vi "Create Events.vi"(0 "Display State In":T2={"Nspeakers"=13, "actions"=[], "Wspeaker"=13, "hover"={"type"=enum."None", "index"=0}, "locked"=FALSE, "states"=[], "sel speak"=13, "selected"=refnum, "Events"={"Selection change"=refnum}}, 9 "Container State":T6, 11 "error in (no error)":errorcluster) -> (4 "Display State Out":T2={"Nspeakers"=13, "actions"=[], "Wspeaker"=13, "hover"={"type"=enum."None", "index"=0}, "locked"=FALSE, "states"=[], "sel speak"=13, "selected"=refnum, "Events"={"Selection change"=refnum}}, 8 "Events":T1, 15 "error out":errorcluster)   [LabVIEW 2015, in "SAC Config.xctl"]
uses:
  SAC Config.xctl
  <vilib>/_xctls/Container State.ctl
  State.vi
  Hover Data.ctl
  Hover Item.ctl
  Speaker State.ctl
  Events.ctl
  Selection changed.ctl
  <vilib>/_xctls/XControlSupport.lvlib
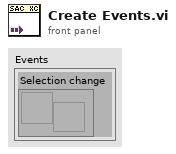
[diagram p1: front panel]
types:
  T1 = typedef "SAC Config.xctl/Events.ctl" = cluster{"Selection change":refnum<user-event>}
  T2 = typedef "SAC Config.xctl/State.vi" = cluster{"Nspeakers":i32, "actions":string[], "Wspeaker":i32, "hover":T3, "locked":bool, "states":T5[], "sel speak":i32, "selected":refnum<vi>, "Events":T1}
  T3 = typedef "SAC Config.xctl/Hover Data.ctl" = cluster{"type":T4, "index":i32}
  T4 = typedef "SAC Config.xctl/Hover Item.ctl" = enum16{"None", "Speaker"}
  T5 = typedef "SAC Config.xctl/Speaker State.ctl" = cluster{"cal":bool, "selected":bool}
  T6 = typedef "XControlSupport.lvlib/Container State.ctl" = cluster{"Indicator?":bool, "Run Mode?":bool, " Refnum":refnum<vi>}
  T7 = typedef "SAC Config.xctl/Selection changed.ctl" = cluster{"Value":i32[]}
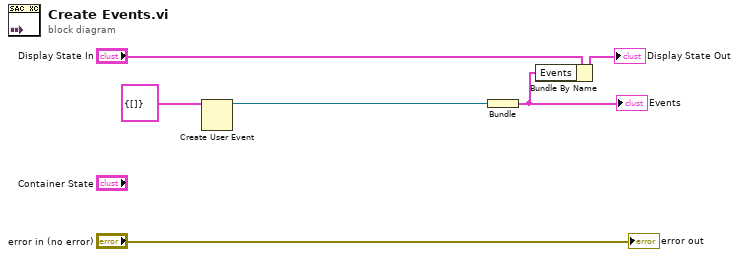
[diagram p0: block diagram]
diagram:
  n1 = Create User Event(user event datatype=T7 {"Value"=[]} ("Event Data")) -> (user event=w2:refnum<user-event>)  [unwired: 1 in, 1 out]
  n2 = Bundle("Event Data"=w2) -> (w1:cluster{"Event Data":refnum<user-event>})  [unwired: 1 in]
  "Events" <- w1
  n3 = Bundle By Name(cluster="Display State In", "Events"=w1) -> (→"Display State Out":T2)
  "error out" <- "error in (no error)"
